vi "Get Network Adapter Settings.vi"(8 "error in (no error)":errorcluster, 11 "Device in":refnum<class "Device.lvclass">=refnum) -> (0 "error out":errorcluster, 2 "Network Adapter Settings":T1[](array[typedef]) {"IP Address Request Mode" items=["Static"=1, "DHCP/Link Local"=2, "Link-Local Only"=4, "DHCP Only"=8]; "Adapter Type" items=["Disabled"=1, "TCP/IP Ethernet"=2, "Deterministic"=4, "EtherCAT"=8, "TCP/IP WLAN Connect"=32, "TCP/IP WLAN Create"=64]; "Adapter Mode" items=["Disabled"=1, "TCP/IP Ethernet"=2, "Deterministic"=4, "EtherCAT"=8, "TCP/IP WLAN Connect"=32, "TCP/IP WLAN Create"=64]}, 3 "Device out":refnum<class "Device.lvclass">)   [LabVIEW 2015]
uses:
  Device.lvclass
  Controls/NetworkAdapterSettings.ctl
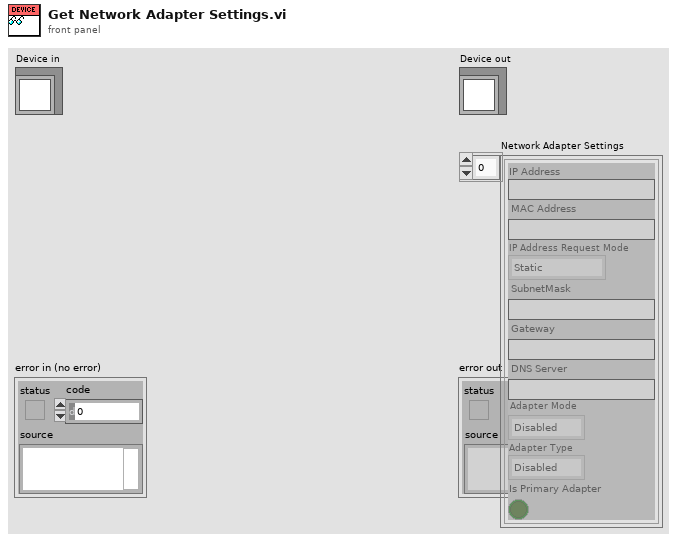
[diagram p1: front panel]
types:
  T1 = typedef "RT Management.lvlib/Device.lvclass/NetworkAdapterSettings.ctl" = cluster{"IP Address":string, "MAC Address":string, "IP Address Request Mode":u32, "SubnetMask":string, "Gateway":string, "DNS Server":string, "Adapter Mode":u32, "Adapter Type":u32, "Is Primary Adapter":bool}
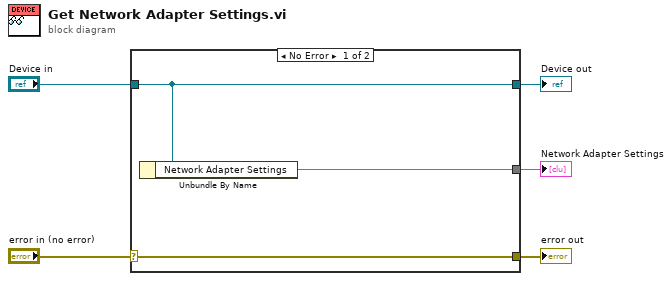
[diagram p0: block diagram]
diagram:
  n1 = case shown="No Error" "error in (no error)" {
    selector: "error in (no error)" -> [w8 w9]
    tunnel: [w8 w9] -> w4
    tunnel: [w7 w10] -> w2
    tunnel: "Device in" -> [w7 w10]
    tunnel: [w6 _] -> w1
    frame No Error {
      n2 = Unbundle By Name(w7) -> ("Network Adapter Settings"=w6)
    }
    frame Error {
    }
  }
  "error out" <- w4
  "Device out" <- w2
  "Network Adapter Settings" <- w1
